vi "MagnetoGUI_Vorschlag.vi"() -> ()   [LabVIEW 2016]
uses:
  controls/GUI Parameter.ctl
  controls/State.ctl
  controls/Data.ctl
panel:
  out "Tab Control":T1(tab)
  in  "Taster Einstellungen":bool
  in  "Anzahl Messpunkte Neukurve":i8=16 min=10 max=30 step=1
  out "Hystereseschleife und Neukurve / Preview":cluster{dbl[], dbl[]}[](graph) caption="XY Graph"
  in  "Plot_Speichern":bool
  out "Status":bool
  in  "Start Button":bool
  in  "Maximieren":bool
  in  "GUI Parameter":T2={"Eisenquerschnitt [mm^2]"=45.0, "Wirksame Länge [cm]"=94.0, "Primärwindungszahl"=700.0, "Sekundärwindungszahl"=700.0, "Messwiderstand [Ohm]"=1.0, "Spannungsteilerverhaeltnis (1/x)"=1.0, "Probenbezeichnung"="", "Dichte des Eisens [g/cm^3]"=7.0, "magn. Flussdichte [T]"=2.0, "Frequenz [Hz]"=50.0, "Namen"="", "Gruppe"=""}
  in  "Neukurve Messen?":bool
  in  "Minimale Spannung [V]":dbl=0.01
  in  "Maximale Spannung [V]":dbl=10.0
  out "Faktor2":dbl
  out "Faktor1":dbl
  out "Theo. Primärwindungszahl":dbl
  in  "Taster Hauptansicht":bool
  in  "VISA Name Oszilloscope":refnum<visa-resource-name>="USB0::0x0957::0x179B::MY54313507::INSTR"
  in  "VISA Name Frequenzgen.":refnum<visa-resource-name>="USB0::0x0957::0x0407::MY44043889::INSTR"
  in  "Anzahl der Oszi-Messpunkte":i32=6000
  in  "Excel Export":bool
  out "Gruppe":string
  out "Namen":string
  out "Frequenz [Hz]":dbl
  out "magn. Flussdichte [T]":dbl
  out "Dichte des Eisens [g/cm^3]":dbl
  out "Probenbezeichnung":string
  out "Spannungsteilerverhältnis (1/x)":dbl
  out "Messwiderstand [Ohm]":dbl
  out "Sekundärwindungszahl":dbl
  out "Primärwindungszahl":dbl
  out "Wirksame Länge [cm]":dbl
  out "Eisenquerschnitt [mm^2]":dbl
  in  "Minimieren":bool
  in  "Ansicht_Speichern":bool
  out "Hystereseschleife und Neukurve":cluster{dbl[], dbl[]}[](graph) caption="XY Graph"
  in  "Plot_Speichern 2":bool
  out "Datum/Uhrzeit":timestamp format="%<%H:%M\n%d/%m/%y>T"
  out "Hystereseverluste [W]":dbl
  # "Laborversuch: Magnetische Eigenschaften"
  # "Laborversuch: Magnetische Eigenschaften"
  # "Oszilloskop Messpunkte"
  # "System Setup"
  # "Frequenzgenerator"
  # "Strombegrenzung"
  # "Anzeige der berechneten Größen"
  # "Maximal Strom [A]"
  # "Laborversuch: Magnetische Eigenschaften"
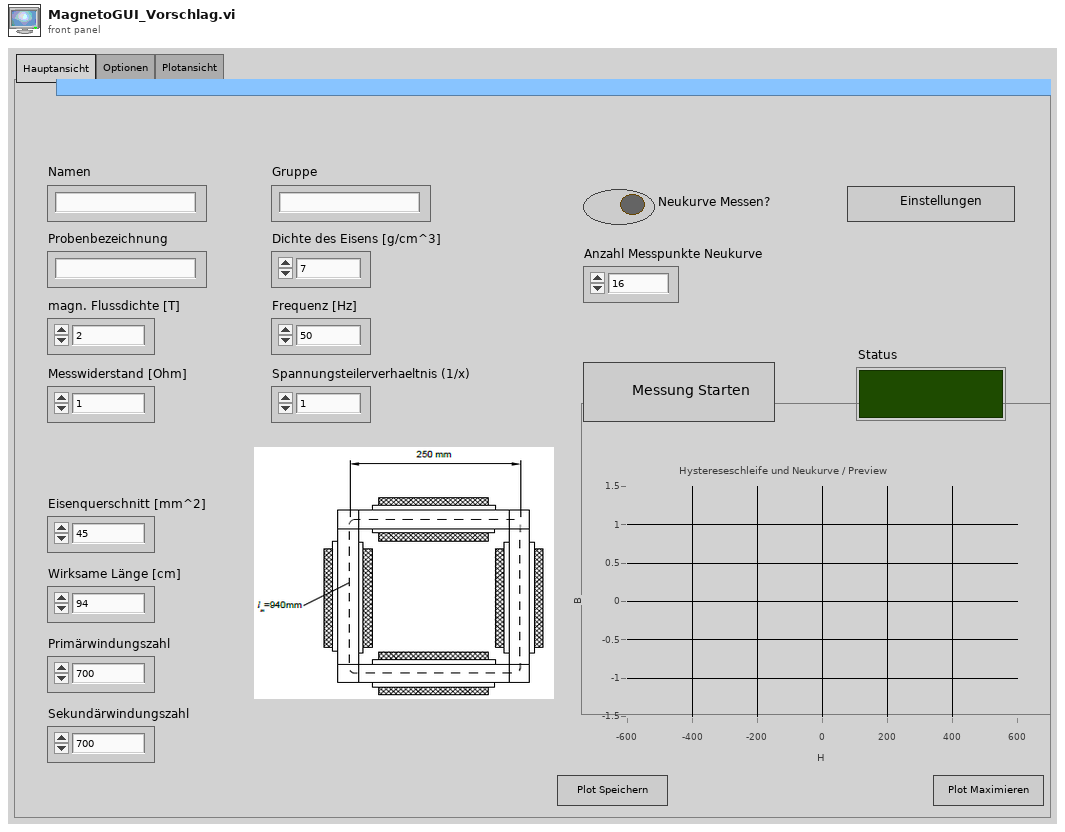
[diagram p1: front panel]
types:
  T1 = enum32{"Hauptansicht", "Optionen", "Plotansicht"}
  T2 = typedef "GUI Parameter.ctl" = cluster{"Eisenquerschnitt [mm^2]":dbl, "Wirksame Länge [cm]":dbl, "Primärwindungszahl":dbl, "Sekundärwindungszahl":dbl, "Messwiderstand [Ohm]":dbl, "Spannungsteilerverhaeltnis (1/x)":dbl, "Probenbezeichnung":string, "Dichte des Eisens [g/cm^3]":dbl, "magn. Flussdichte [T]":dbl, "Frequenz [Hz]":dbl, "Namen":string, "Gruppe":string}
  T3 = typedef "Data.ctl" = cluster{"GUI Einstellungen":cluster{"Spannungsabweichung":dbl, "Maximale Spannung FG":dbl, "Faktor1":dbl, "Faktor2":dbl, "Theoretische Primärwindungszahl":dbl, "Anzahl der Messpunkte":i32, "VISA Name Oszilloscope":refnum<visa-resource-name>, "VISA Name Frequenzgenerator":refnum<visa-resource-name>, "Minimale Spannung FG":dbl, "Pfad für Messwerte und Plots":path}, "GUI data":cluster{"Eisenquerschnitt [mm^2]":dbl, "Wirksame Länge [cm]":dbl, "Primärwindungszahl":dbl, "Sekundärwindungszahl":dbl, "Messwiderstand [Ohm]":dbl, "Spannungsteilerverhaeltnis (1/x)":dbl, "Probenbezeichnung":string, "Dichte des Eisens [g/cm^3]":dbl, "magn. Flussdichte [T]":dbl, "Frequenz [Hz]":dbl, "Namen":string, "Gruppe":string}, "B - Neukurve Array":dbl[], "H - Neukurve Array":dbl[], "Messung Hystereseschleife":cluster{"b_gew":dbl, "b_kor":dbl, "hys_verluste":dbl, "punkte":i32, "B - Hysterese Array":dbl[], "H - Hysterese Array":dbl[]}, "Messung Neukurve":cluster{"Neukurve Messen?":bool, "Anzahl Messpunkte Neukurve":i8}, "Globale Variablen":cluster{"merker1":bool, "merker2":bool, "merker3":bool, "merker4":bool, "merker5":bool, "merker6":bool, "merker7":bool, "merker8":bool, "merker9":bool, "bmax1":dbl, "bmin1":dbl, "bmax2":dbl, "bmin2":dbl, "spg_abw":dbl, "Tatsächliche Flussdichte":dbl, "Tatsächliche Anzahl Punkte":dbl, "hmax1":dbl, "hmin1":dbl, "hmax2":dbl}}
  T4 = typedef "State.ctl" = enum16{"Initialisieren", "Warten auf Event", "Starten der Messung", "Initialisieren Hardware", "Flussdichte Einstellen", "Chk Flussdichte Anpassung", "Messung Hystereseschleife", "Entmagnetisieren", "Messung Neukurve", "Messung Kommutierungskurve", "Ausgabe Diagramm", "Ende", "Plot aufnehmen", "Ansicht speichern", "Excel Export"}
  T5 = cluster{"Spannungsabweichung":dbl, "Maximale Spannung FG":dbl, "Faktor1":dbl, "Faktor2":dbl, "Theoretische Primärwindungszahl":dbl, "Anzahl der Messpunkte":i32, "VISA Name Oszilloscope":refnum<visa-resource-name>, "VISA Name Frequenzgenerator":refnum<visa-resource-name>, "Minimale Spannung FG":dbl, "Pfad für Messwerte und Plots":path}
  T6 = cluster{"Eisenquerschnitt [mm^2]":dbl, "Wirksame Länge [cm]":dbl, "Primärwindungszahl":dbl, "Sekundärwindungszahl":dbl, "Messwiderstand [Ohm]":dbl, "Spannungsteilerverhaeltnis (1/x)":dbl, "Probenbezeichnung":string, "Dichte des Eisens [g/cm^3]":dbl, "magn. Flussdichte [T]":dbl, "Frequenz [Hz]":dbl, "Namen":string, "Gruppe":string}
  T7 = cluster{"merker1":bool, "merker2":bool, "merker3":bool, "merker4":bool, "merker5":bool, "merker6":bool, "merker7":bool, "merker8":bool, "merker9":bool, "bmax1":dbl, "bmin1":dbl, "bmax2":dbl, "bmin2":dbl, "spg_abw":dbl, "Tatsächliche Flussdichte":dbl, "Tatsächliche Anzahl Punkte":dbl, "hmax1":dbl, "hmin1":dbl, "hmax2":dbl}
  T8 = cluster{"b_gew":dbl, "b_kor":dbl, "hys_verluste":dbl, "punkte":i32, "B - Hysterese Array":dbl[], "H - Hysterese Array":dbl[]}
  T9 = cluster{"H - Hysterese Array":dbl[], "B - Hysterese Array":dbl[]}
  T10 = cluster{"H - Neukurve Array":dbl[], "B - Neukurve Array":dbl[]}
  T11 = cluster{"H - Neukurve Array":dbl[], "B - Neukurve Array":dbl[]}[]
  T12 = typedef "imagedata.ctl" = cluster{"image type":i32, "image depth":i32, "image":u8[], "mask":u8[], "colors":u32[], "Rectangle":cluster{"left":i16, "top":i16, "right":i16, "bottom":i16}}
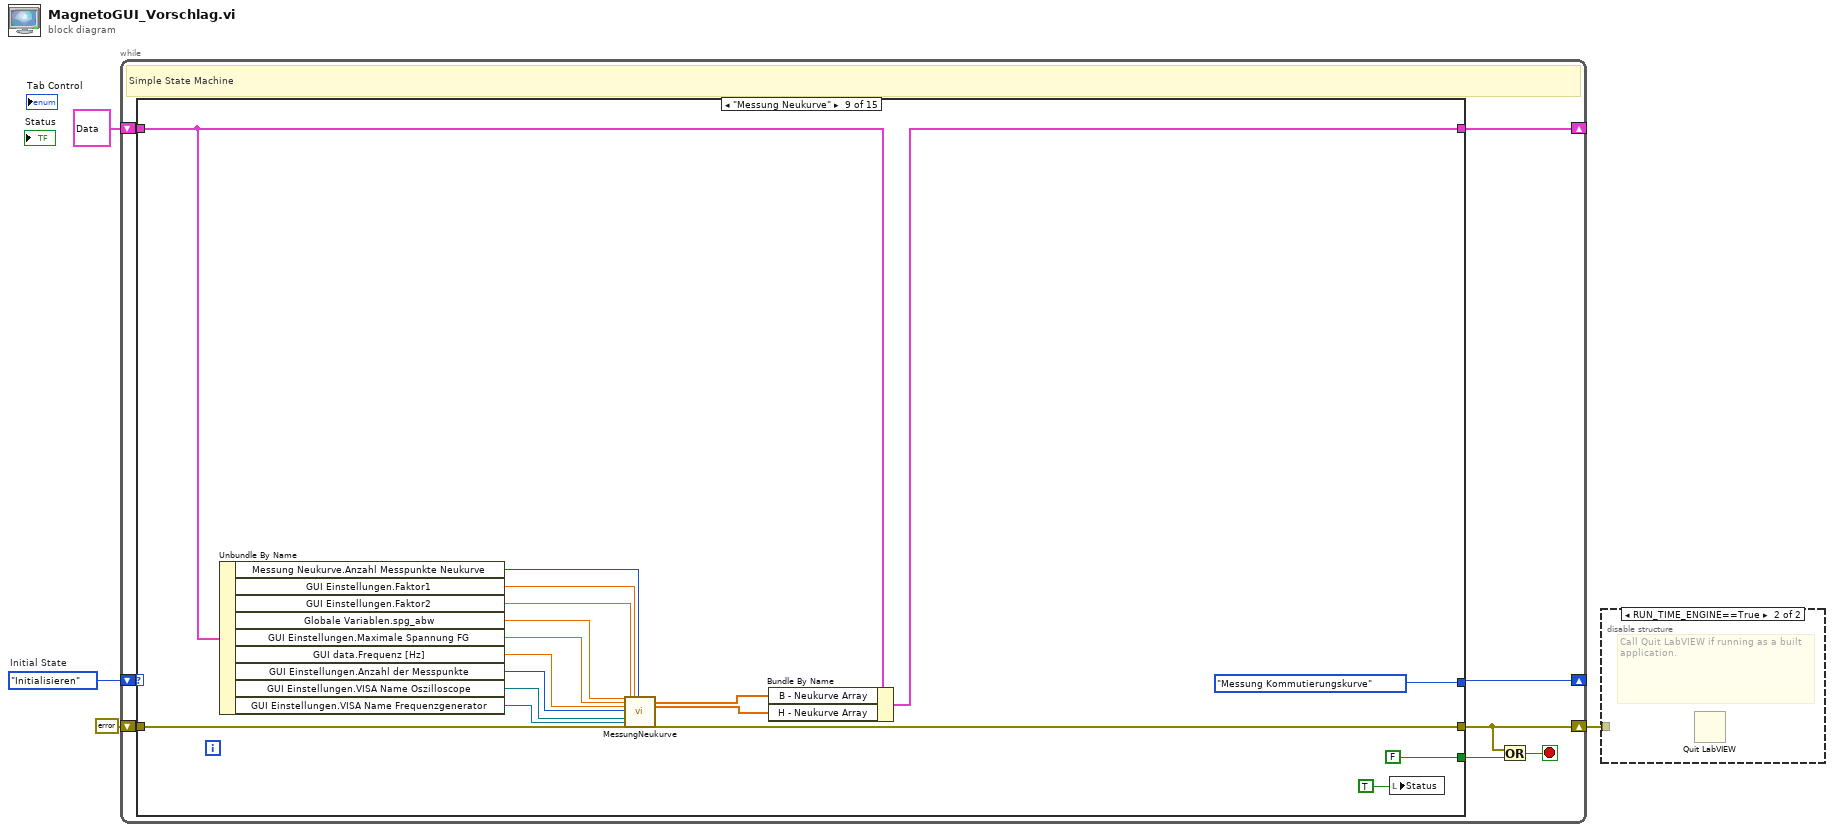
[diagram p0: block diagram]
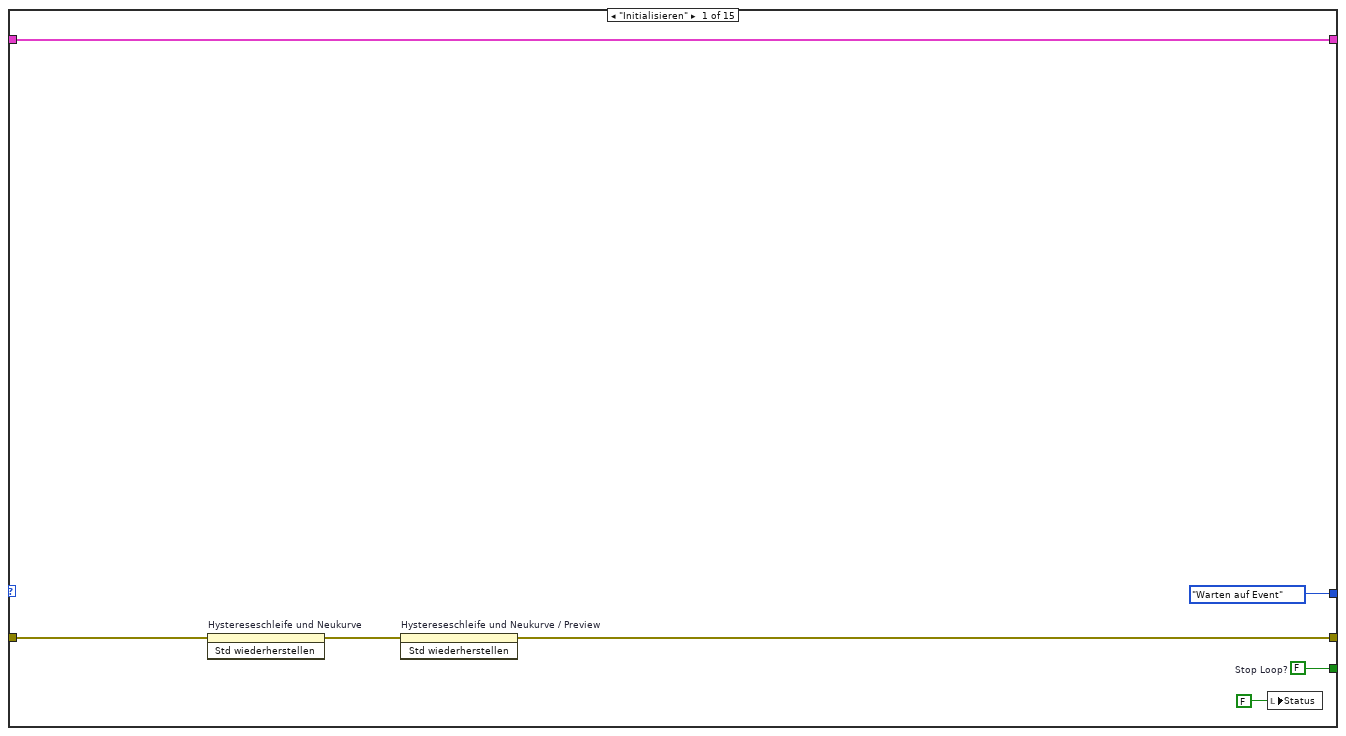
[diagram p2: hidden frame]
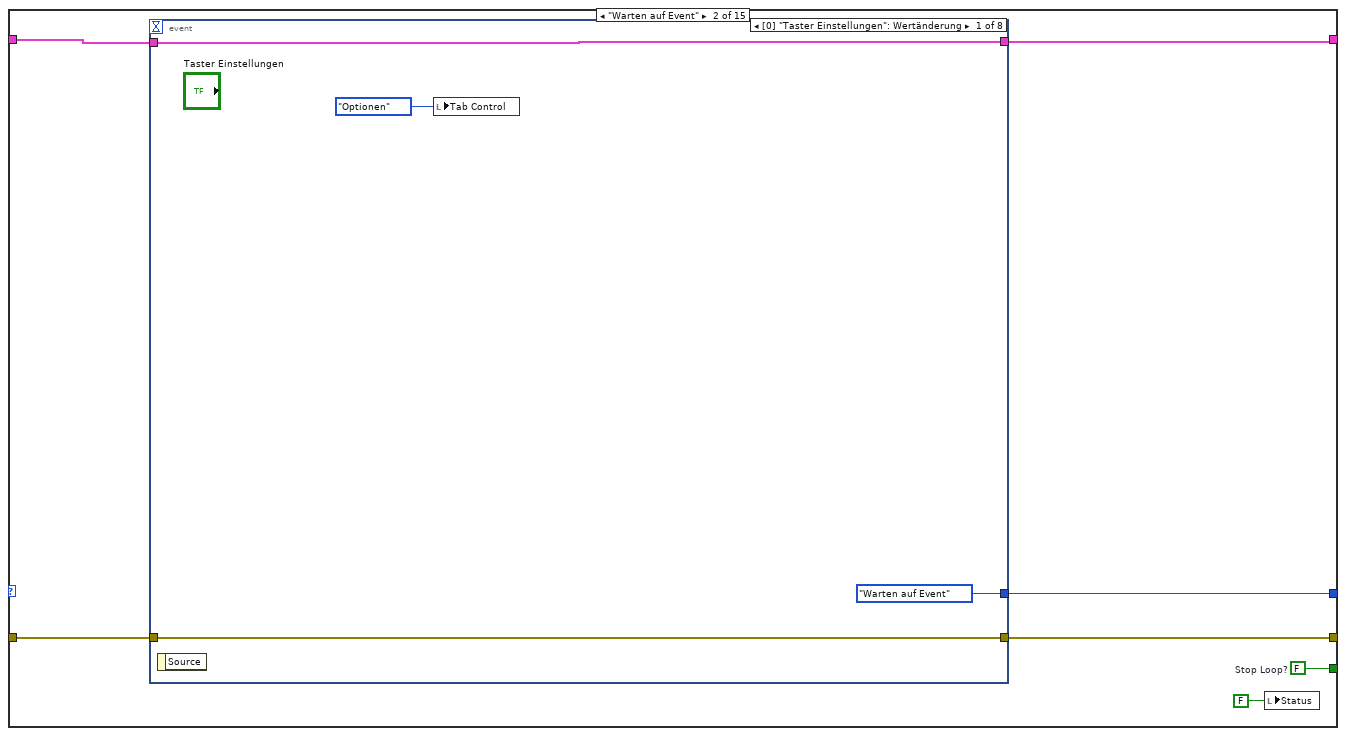
[diagram p3: hidden frame]
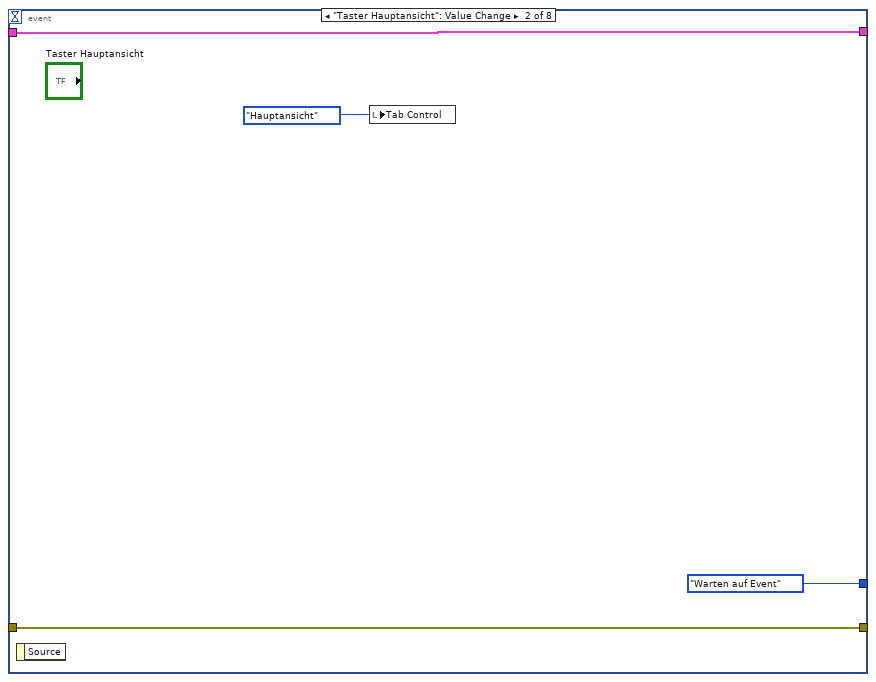
[diagram p4: hidden frame]
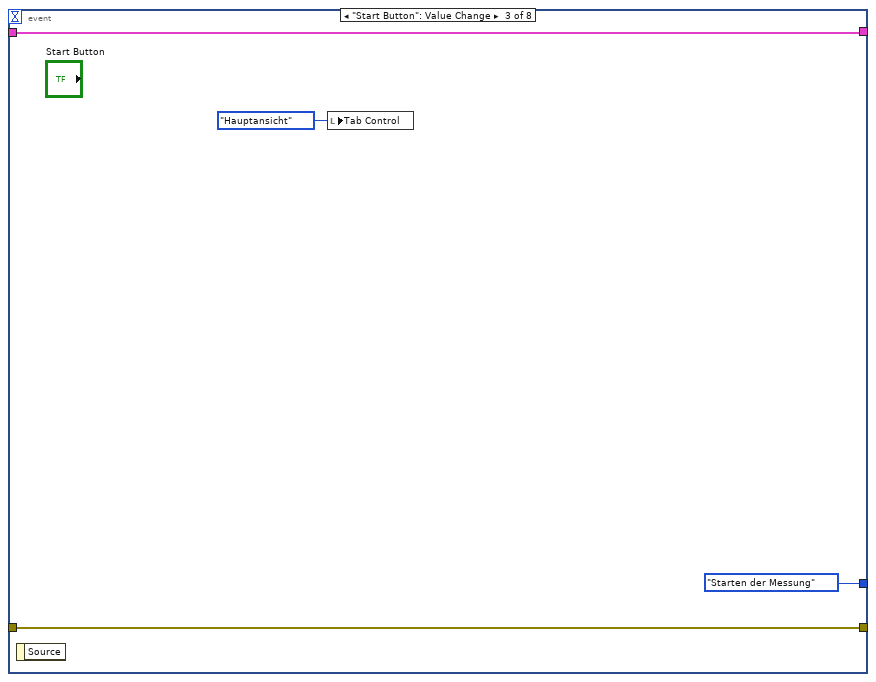
[diagram p5: hidden frame]
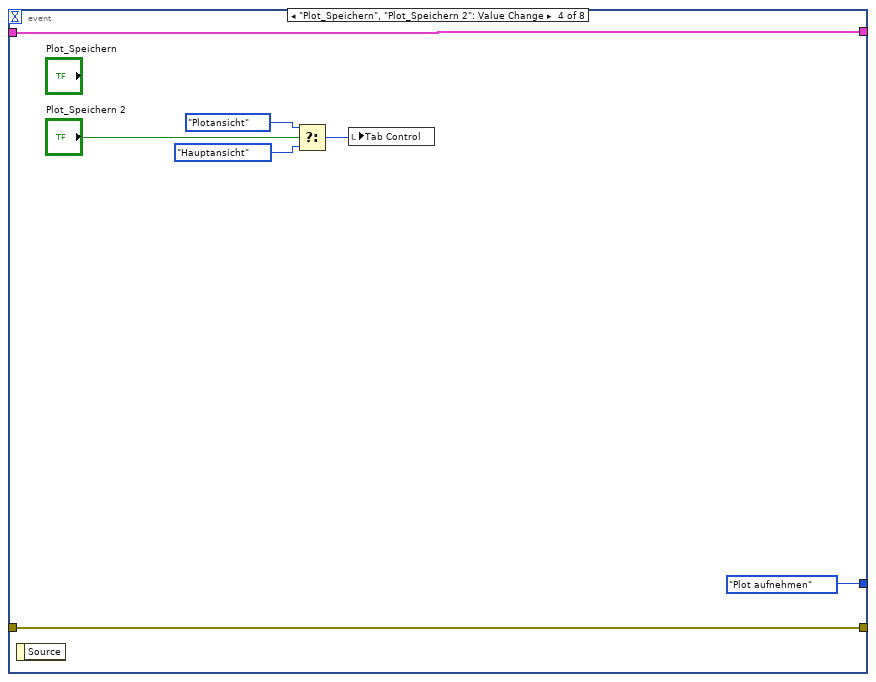
[diagram p6: hidden frame]
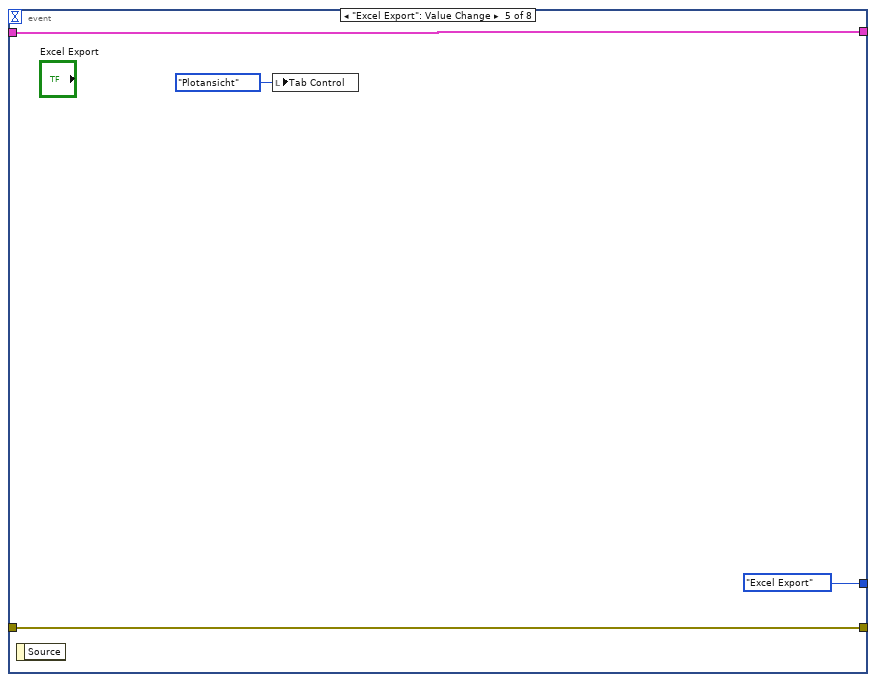
[diagram p7: hidden frame]
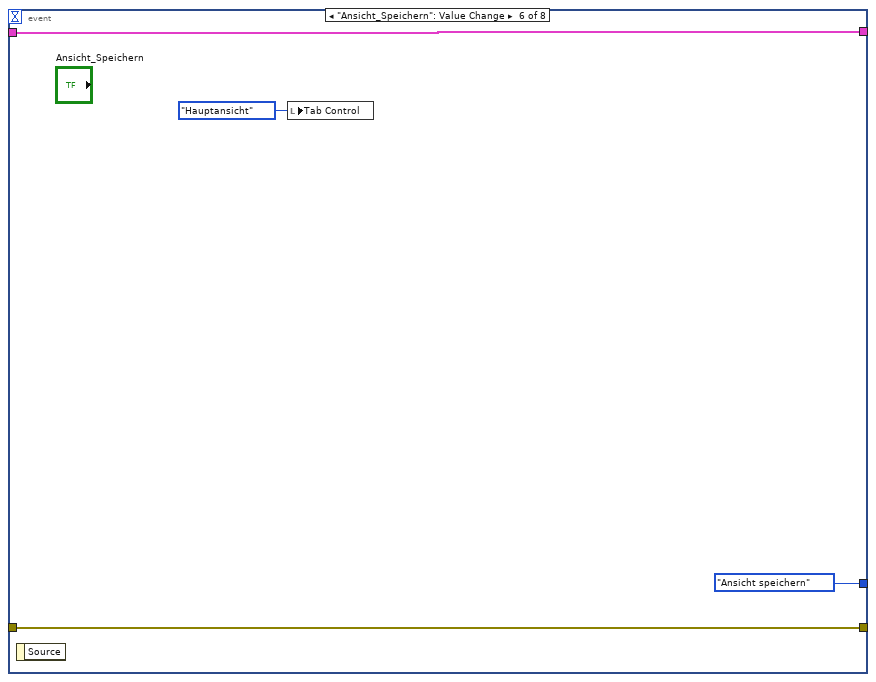
[diagram p8: hidden frame]
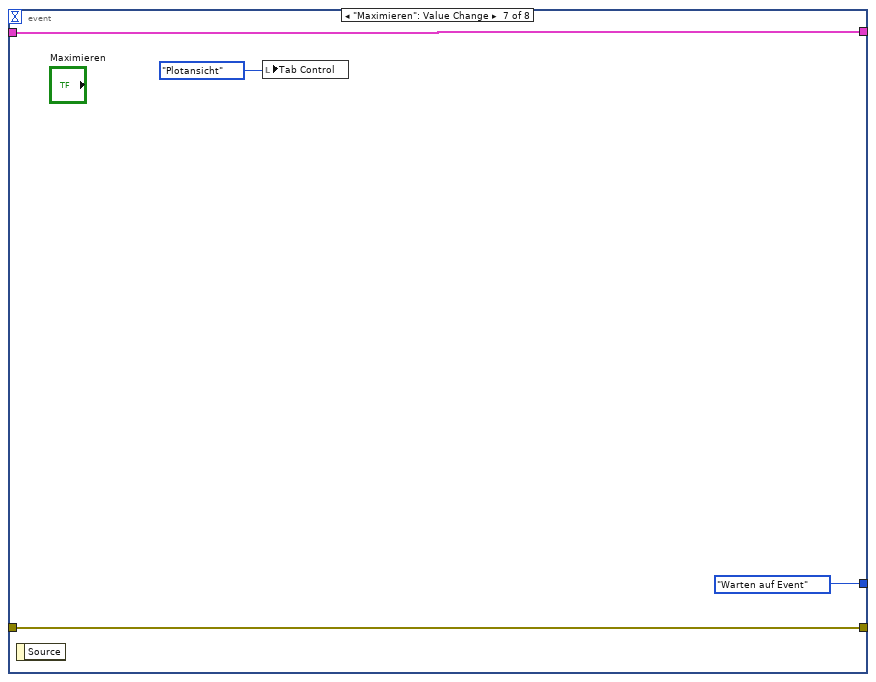
[diagram p9: hidden frame]
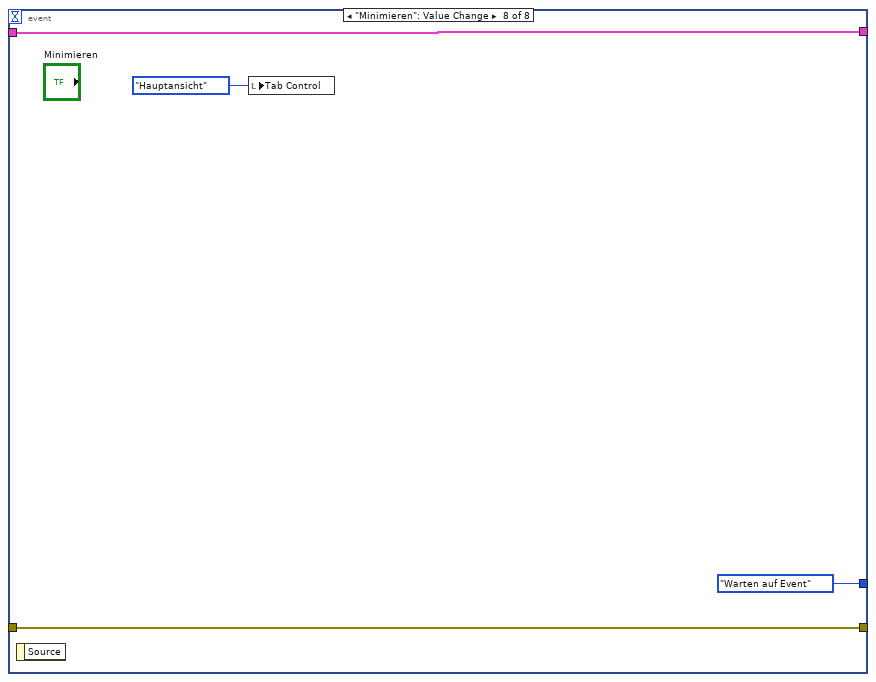
[diagram p10: hidden frame]
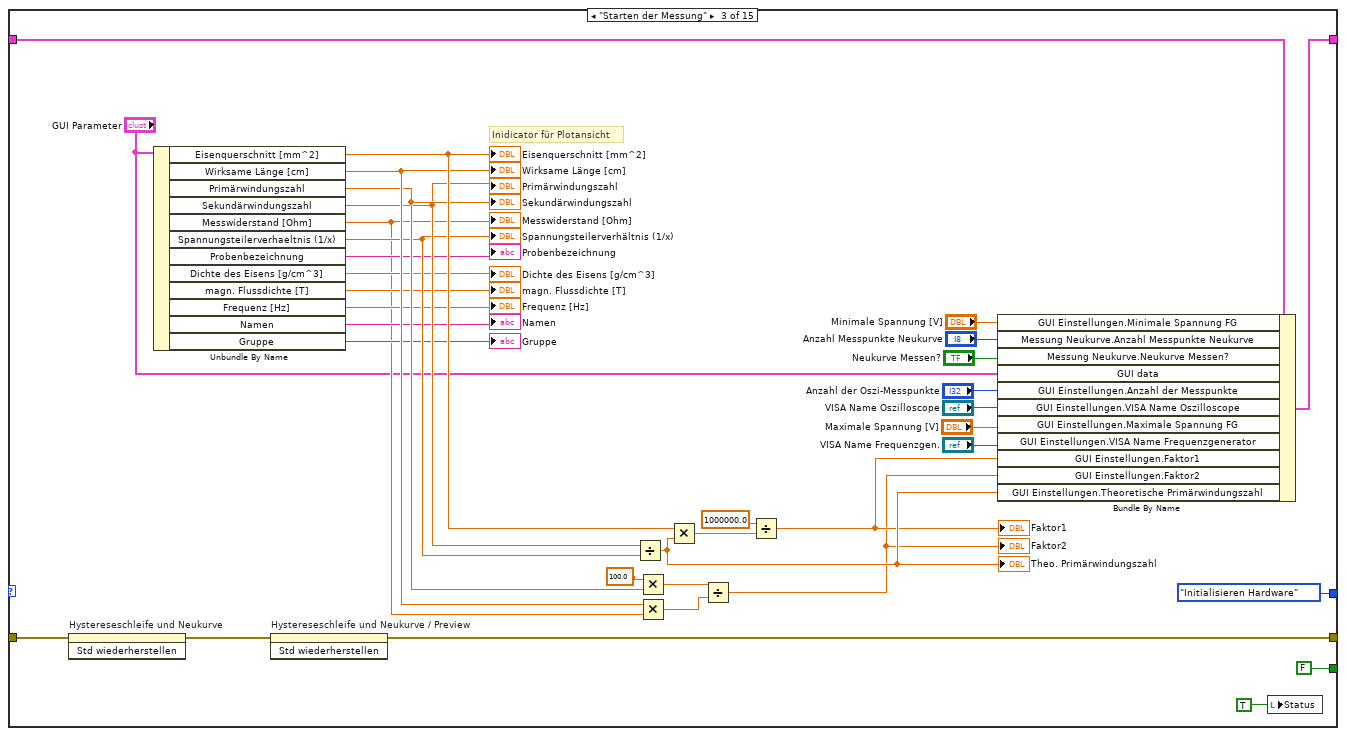
[diagram p11: hidden frame]
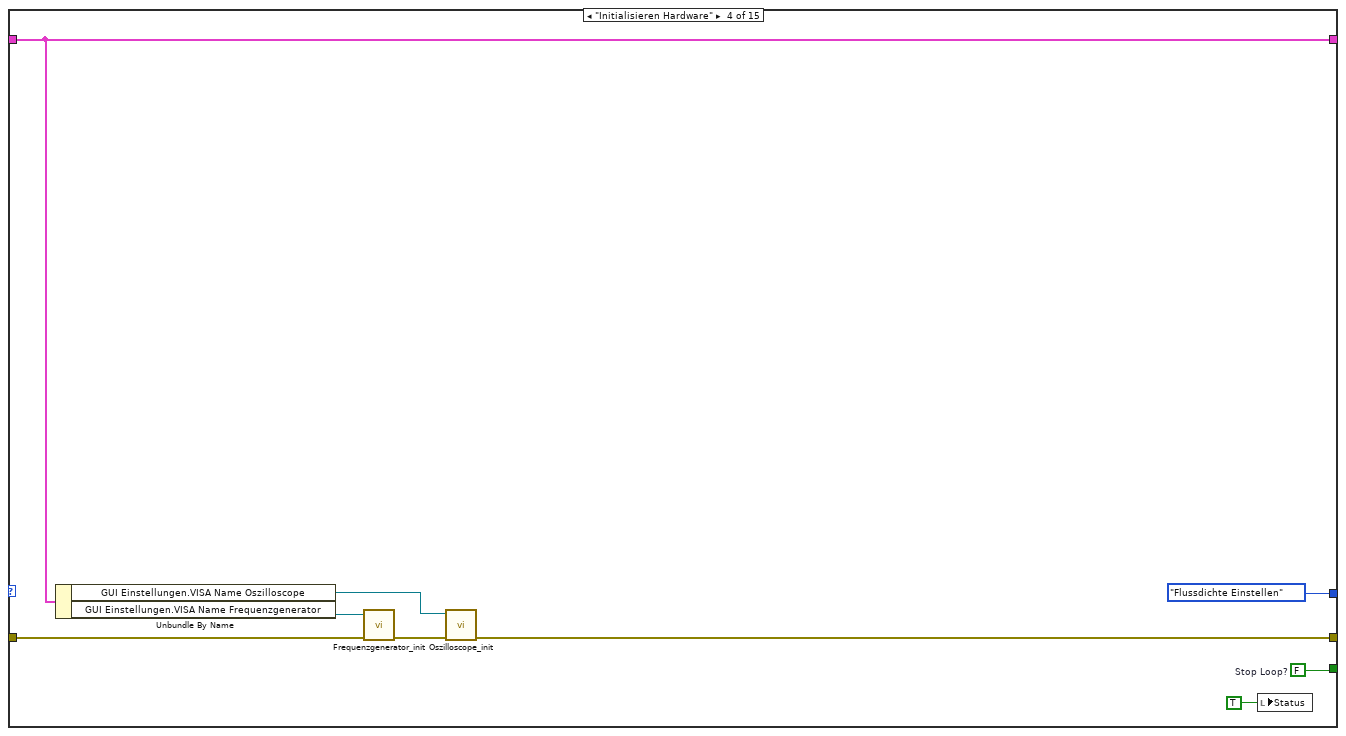
[diagram p12: hidden frame]
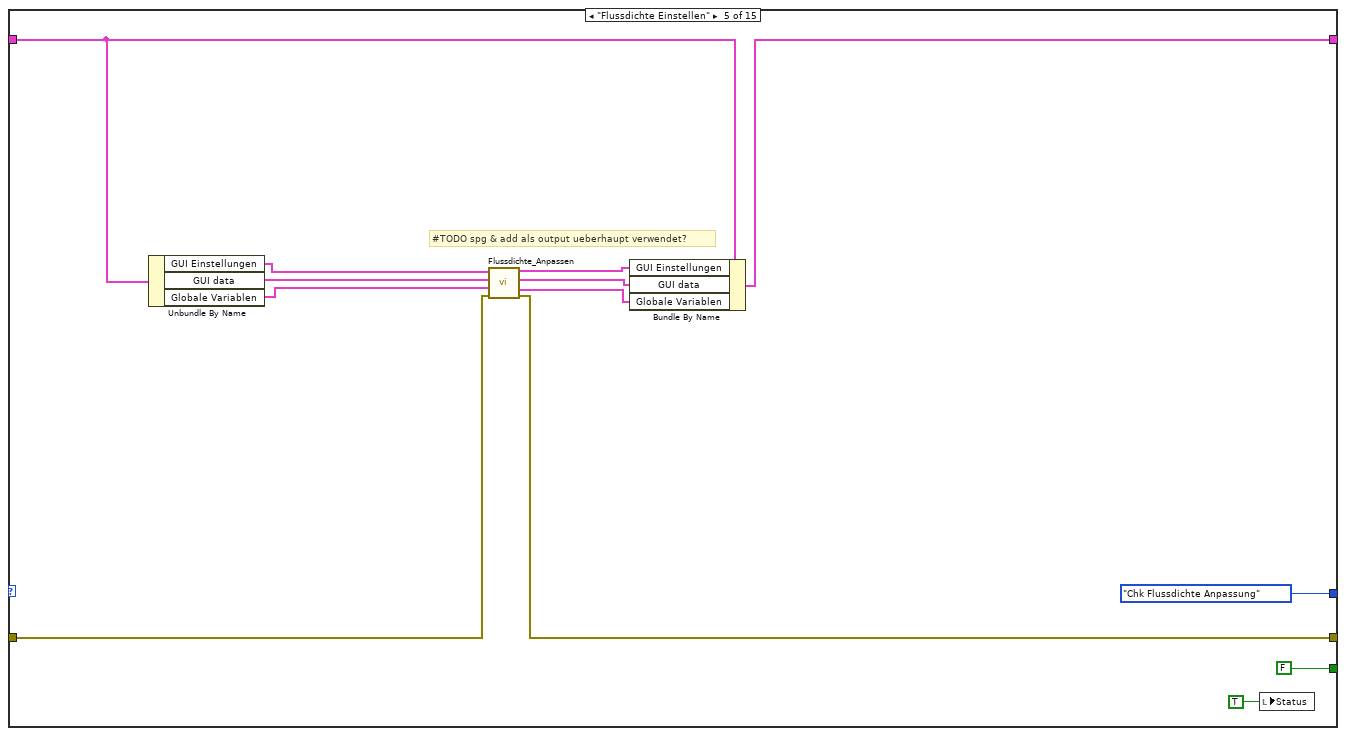
[diagram p13: hidden frame]
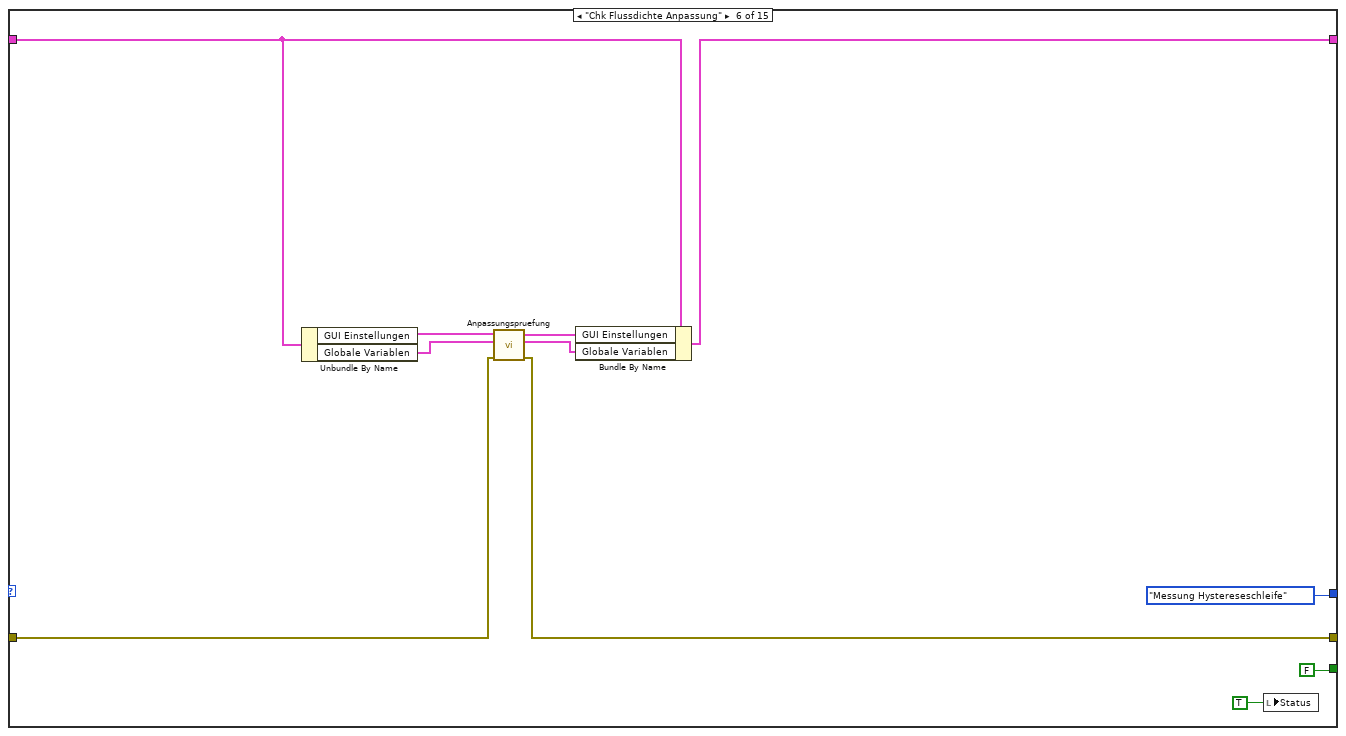
[diagram p14: hidden frame]
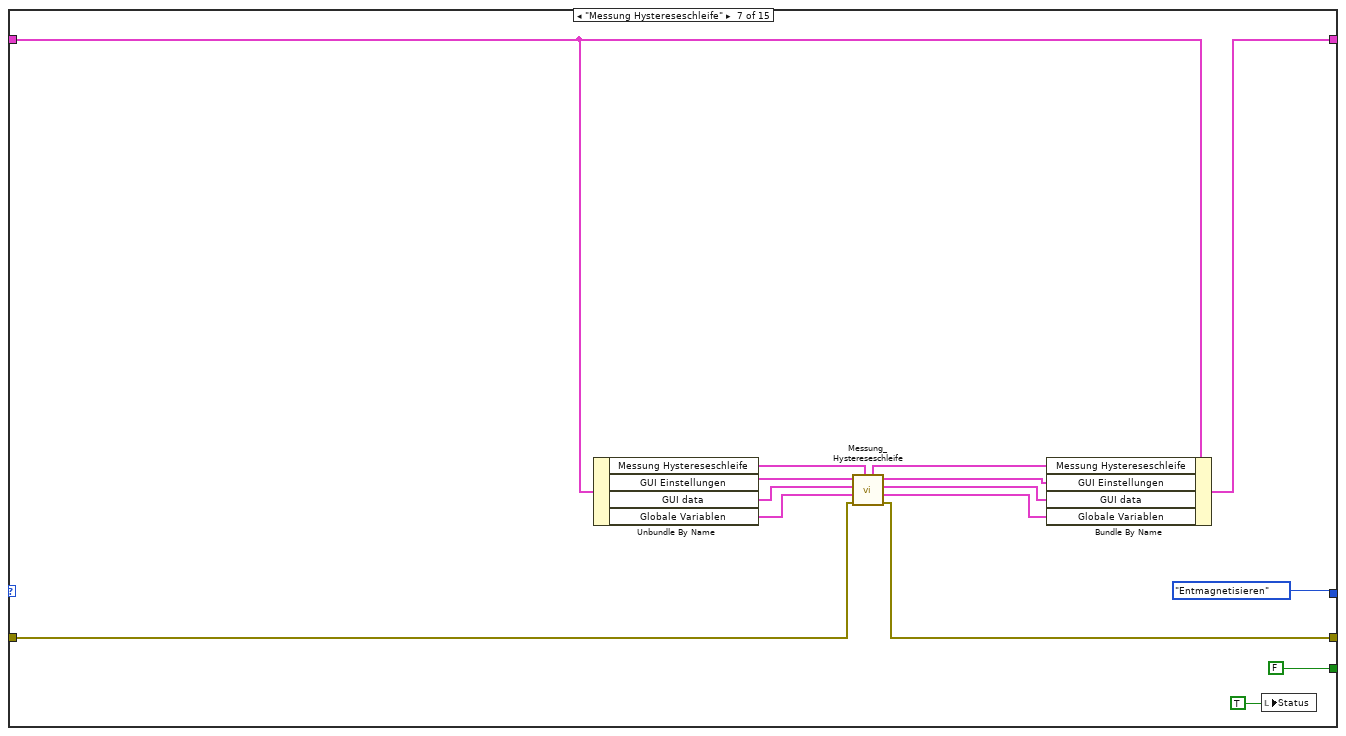
[diagram p15: hidden frame]
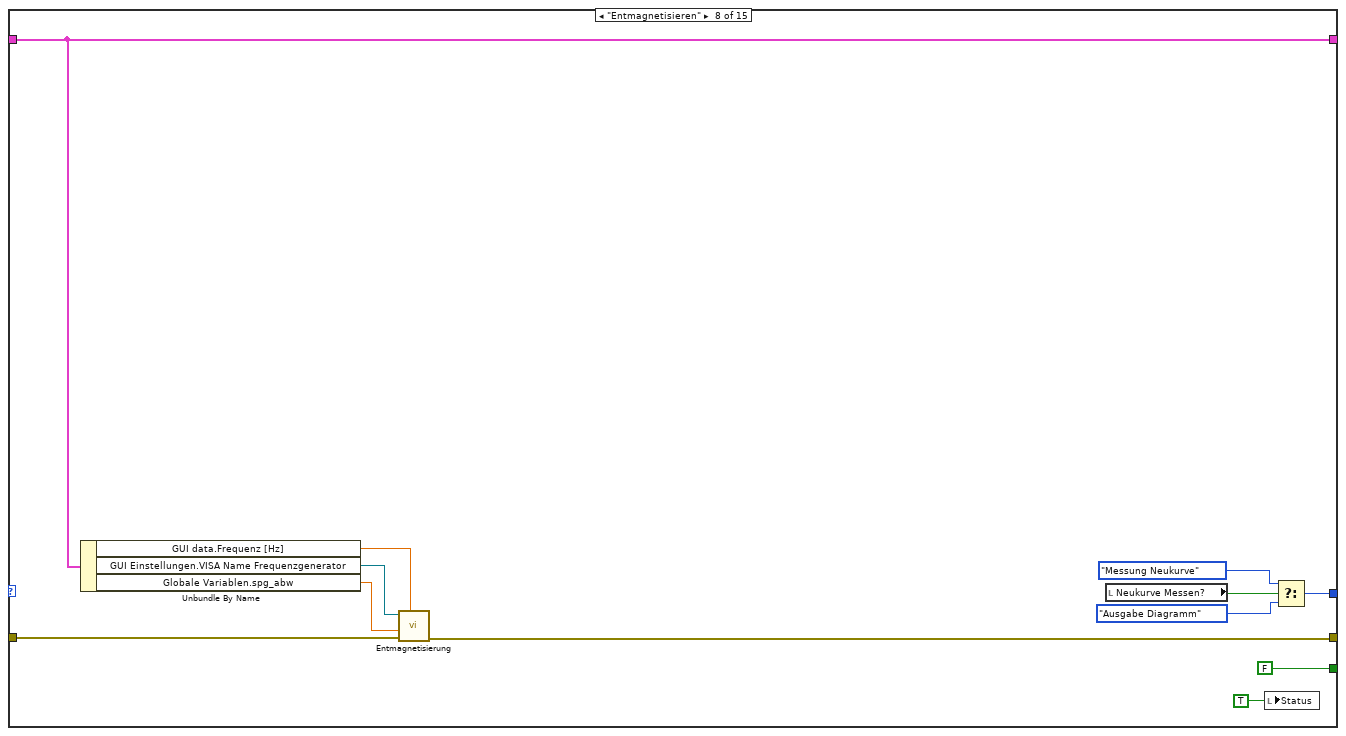
[diagram p16: hidden frame]
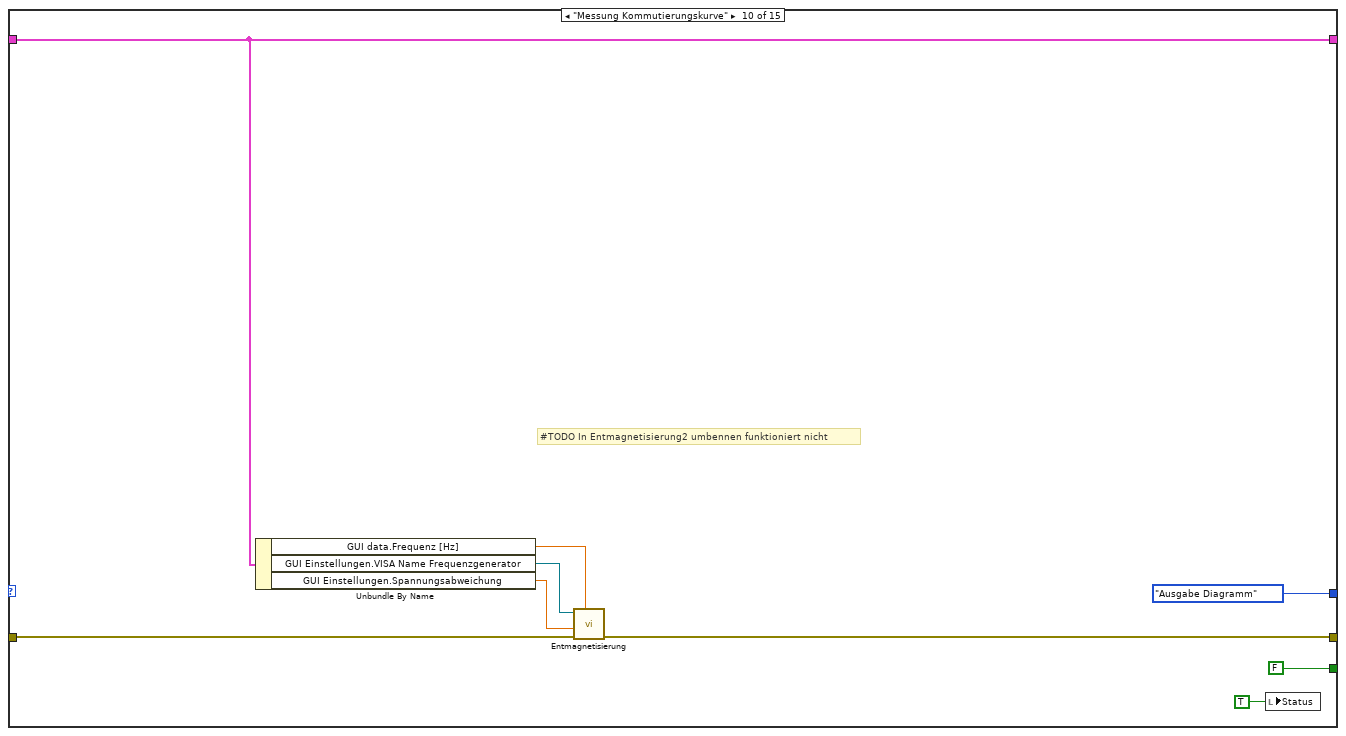
[diagram p17: hidden frame]
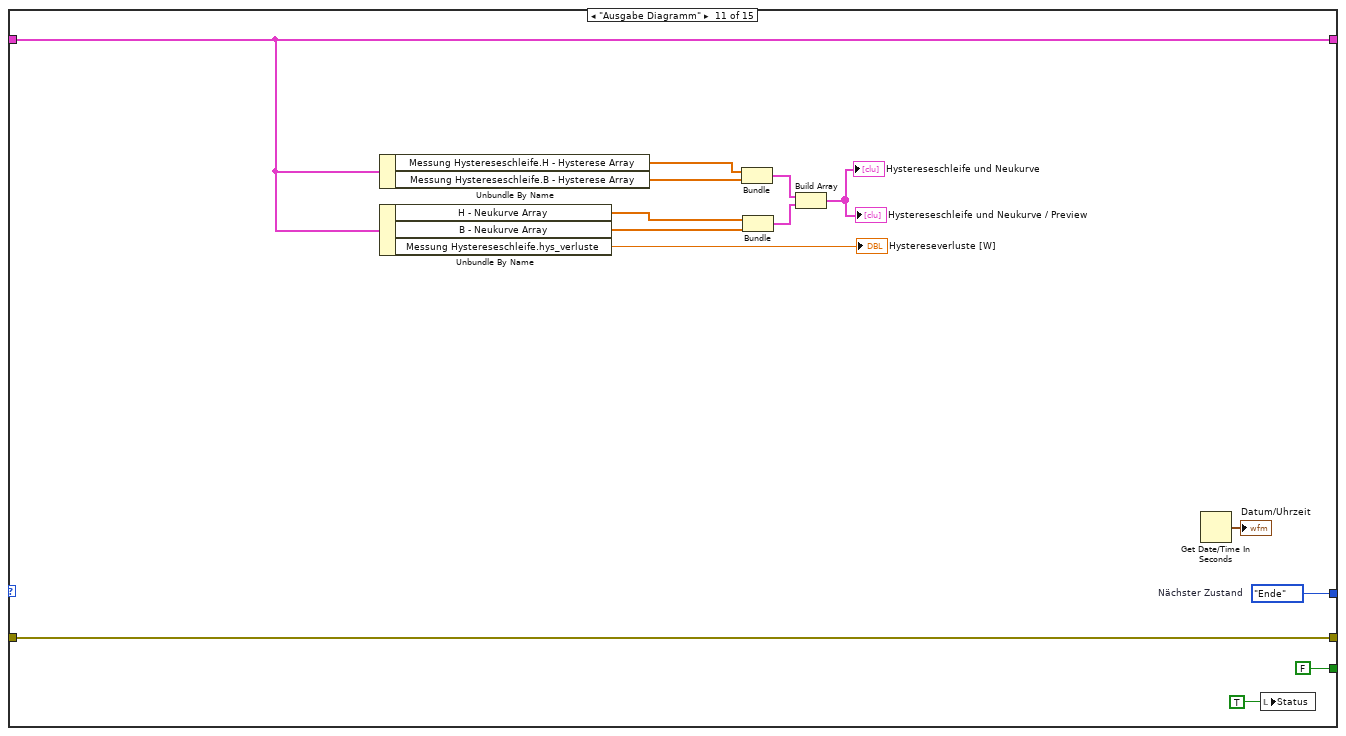
[diagram p18: hidden frame]
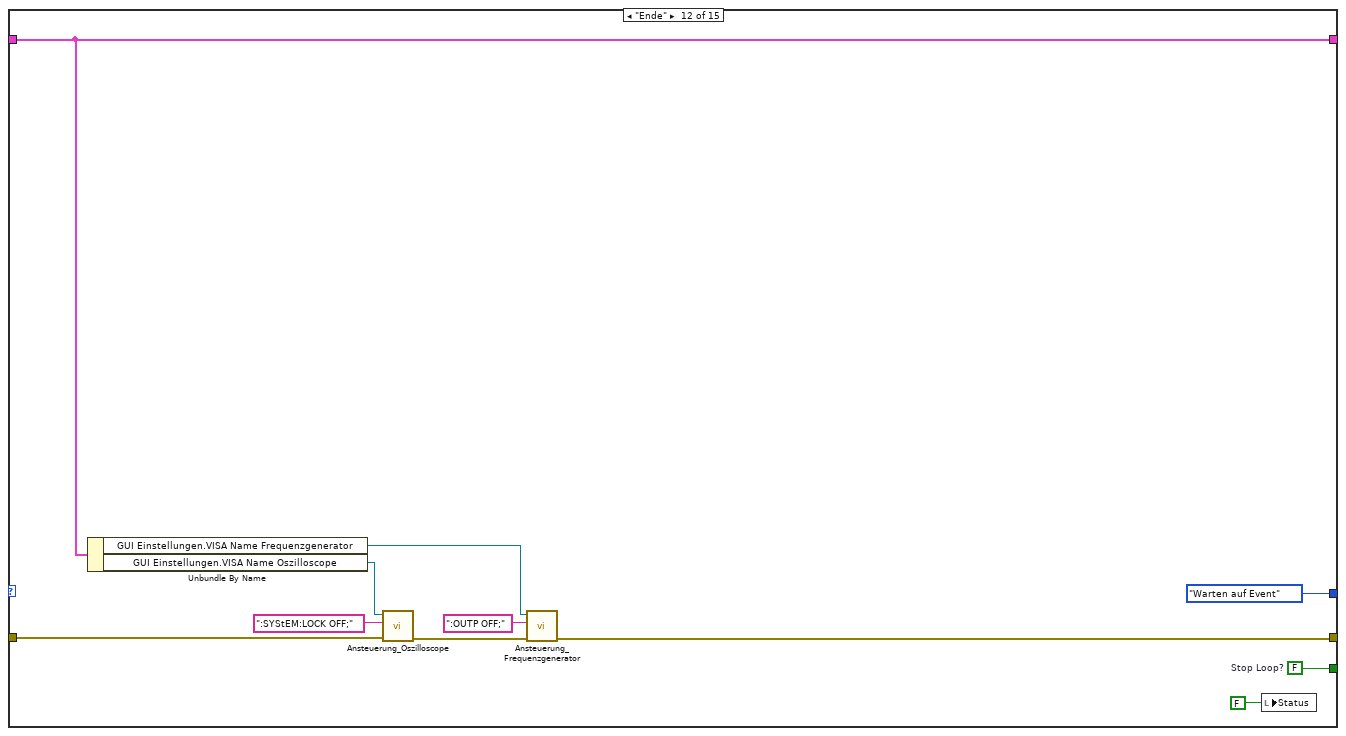
[diagram p19: hidden frame]
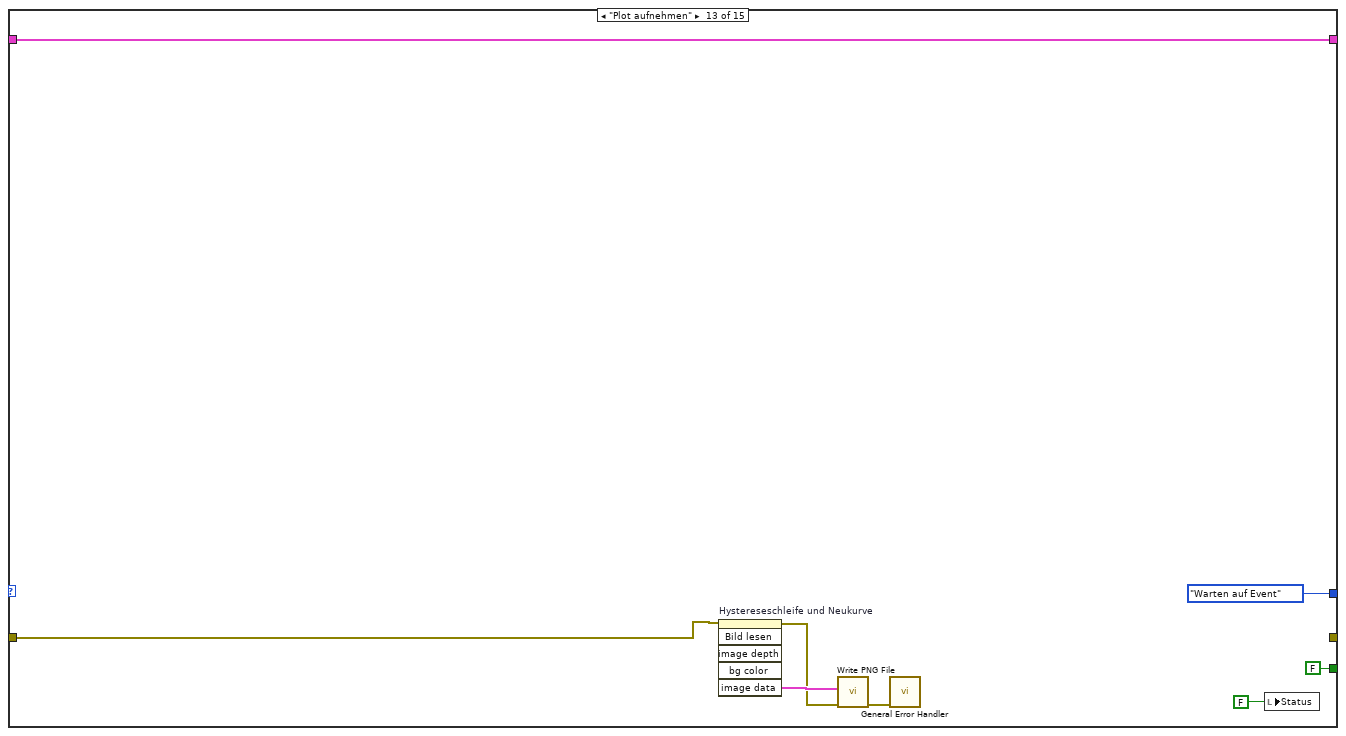
[diagram p20: hidden frame]
diagram:
  w4 = State."Initialisieren"  # Initial State
  n1 = while {
    shift-right: [w11] -> _
    shift-left: w4 -> [w12]
    shift-right: [w9] -> _
    shift-left: T3 {"GUI Einstellungen"={"Spannungsabweichung"=0.0, "Maximale Spannung FG"=0.0, "Faktor1"=0.0, "Faktor2"=0.0, "Theoretische Primärwindungszahl"=0.0, "Anzahl der Messpunkte"=0, "VISA Name Oszilloscope"="", "VISA Name Frequenzgenerator"="", "Minimale Spannung FG"=0.0, "Pfad für Messwerte und Plots"=path ""}, "GUI data"={"Eisenquerschnitt [mm^2]"=0.0, "Wirksame Länge [cm]"=0.0, "Primärwindungszahl"=0.0, "Sekundärwindungszahl"=0.0, "Messwiderstand [Ohm]"=0.0, "Spannungsteilerverhaeltnis (1/x)"=0.0, "Probenbezeichnung"="", "Dichte des Eisens [g/cm^3]"=0.0, "magn. Flussdichte [T]"=0.0, "Frequenz [Hz]"=0.0, "Namen"="", "Gruppe"=""}, "B - Neukurve Array"=[], "H - Neukurve Array"=[], "Messung Hystereseschleife"={"b_gew"=0.0, "b_kor"=0.0, "hys_verluste"=0.0, "punkte"=0, "B - Hysterese Array"=[0.0, 0.0], "H - Hysterese Array"=[0.0, 0.0]}, "Messung Neukurve"={"Neukurve Messen?"=FALSE, "Anzahl Messpunkte Neukurve"=16}, "Globale Variablen"={"merker1"=FALSE, "merker2"=FALSE, "merker3"=FALSE, "merker4"=FALSE, "merker5"=FALSE, "merker6"=FALSE, "merker7"=FALSE, "merker8"=FALSE, "merker9"=FALSE, "bmax1"=0.0, "bmin1"=0.0, "bmax2"=0.0, "bmin2"=0.0, "spg_abw"=0.0, "Tatsächliche Flussdichte"=0.0, "Tatsächliche Anzahl Punkte"=0.0, "hmax1"=0.0, "hmin1"=0.0, "hmax2"=0.0}} ("Data") -> [w10]
    shift-right: [w5] -> w1
    shift-left: errorcluster {"status"=FALSE, "code"=0, "source"=""} ("error constant") -> [w8]
    stop <- w6 stop-if-true
    # "Simple State Machine"
    n2 = case shown="\"Messung Neukurve\"" w12 {
      tunnel: [State."Warten auf Event" ("Next State") w26 State."Initialisieren Hardware" ("Next State") State."Flussdichte Einstellen" ("Next State") State."Chk Flussdichte Anpassung" ("Next  State") State."Messung Hystereseschleife" ("Next  State") State."Entmagnetisieren" ("(Value Not Used)") w147 State."Messung Kommutierungskurve" ("(Value Not Used)") State."Ausgabe Diagramm" ("(Value Not Used)") w196 State."Warten auf Event" ("Next  State") State."Warten auf Event" ("Next  State") State."Warten auf Event" ("Next  State") State."Warten auf Event" ("Next  State")] -> w11
      tunnel: [w18 w25 FALSE ("Stop Loop?") w99 FALSE ("Stop Loop?") FALSE ("Stop Loop?") FALSE ("Stop Loop?") FALSE ("Stop Loop?") FALSE ("Stop Loop?") FALSE ("Stop Loop?") FALSE ("Stop Loop?") w209 FALSE ("Stop Loop?") FALSE ("Stop Loop?") FALSE ("Stop Loop?")] -> w7
      tunnel: w10 -> [w17 w24 w75 w105 w114 w126 w133 w156 w163 w177 w191 w207 w217 w225 w232]
      tunnel: [w17 w23 w76 w105 w113 w125 w144 w156 w167 w177 w191 w207 w217 w225 w232] -> w9
      tunnel: w8 -> [w16 w22 w95 w104 w115 w121 w132 w155 w173 w179 w195 w208 w215 w221 w230]
      tunnel: [w14 w21 w77 w102 w109 w122 w134 w154 w172 w178 w195 w202 _ _ w229] -> w5
      frame "Initialisieren" {
        w18 = FALSE  # Stop Loop?
        n3 = invoke on="Hystereseschleife und Neukurve" class="XYGraph (strikt)" method="Std wiederherstellen"(error in=w16) -> (error out=w15:errorcluster)  [unwired: 2 in, 2 out]
        n4 = invoke on="Hystereseschleife und Neukurve / Preview" class="XYGraph (strikt)" method="Std wiederherstellen"(error in=w15) -> (error out=w14:errorcluster)  [unwired: 2 in, 2 out]
        n5 = local write "Status"(FALSE ("Status")) -> ()
      }
      frame "Warten auf Event" {
        w25 = FALSE  # Stop Loop?
        n6 = event shown="[0] \"Taster Einstellungen\": Wertänderung" {
          selector: _ -> [_ _ _ _ _ _ _ _]
          dyn-events: _ -> [_ _ _ _ _ _ _ _]
          timeout: _ -> [_ _ _ _ _ _ _ _]
          tunnel: [State."Warten auf Event" State."Warten auf Event" ("Next State") State."Starten der Messung" ("Next State") State."Plot aufnehmen" ("Next State") State."Excel Export" ("Next State") State."Ansicht speichern" ("Next State") State."Warten auf Event" ("Next State") State."Warten auf Event" ("Next State")] -> w26
          tunnel: w24 -> [w30 w34 w36 w45 w49 w53 w55 w61]
          tunnel: [w30 w34 w36 w45 w49 w53 w55 w61] -> w23
          tunnel: w22 -> [w29 w33 w37 w39 w46 w50 w56 w60]
          tunnel: [w29 w33 w37 w39 w46 w50 w56 w60] -> w21
          event "Taster Einstellungen": Value Change {
            n7 = event-data() -> ()  [unwired: 1 in, 1 out]
            n8 = local write "Tab Control"(T1."Optionen" ("Tab Control")) -> ()
          }
          event "Taster Hauptansicht": Value Change {
            n9 = event-data() -> ()  [unwired: 1 in, 1 out]
            n10 = local write "Tab Control"(T1."Hauptansicht" ("Tab Control")) -> ()
          }
          event "Start Button": Value Change {
            n11 = event-data() -> ()  [unwired: 1 in, 1 out]
            n12 = local write "Tab Control"(T1."Hauptansicht" ("Tab Control")) -> ()
          }
          event "Plot_Speichern", "Plot_Speichern 2": Value Change {
            n13 = event-data() -> ()  [unwired: 1 in, 1 out]
            n14 = Select(t=T1."Plotansicht" ("Tab Control"), s="Plot_Speichern 2", f=T1."Hauptansicht" ("Tab Control")) -> (s? t:f=w40:T1)
            n15 = local write "Tab Control"(w40) -> ()
          }
          event "Excel Export": Value Change {
            n16 = event-data() -> ()  [unwired: 1 in, 1 out]
            n17 = local write "Tab Control"(T1."Plotansicht" ("Tab Control")) -> ()
          }
          event "Ansicht_Speichern": Value Change {
            n18 = event-data() -> ()  [unwired: 1 in, 1 out]
            n19 = local write "Tab Control"(T1."Hauptansicht" ("Tab Control")) -> ()
          }
          event "Maximieren": Value Change {
            n20 = event-data() -> ()  [unwired: 1 in, 1 out]
            n21 = local write "Tab Control"(T1."Plotansicht" ("Tab Control")) -> ()
          }
          event "Minimieren": Value Change {
            n22 = event-data() -> ()  [unwired: 1 in, 1 out]
            n23 = local write "Tab Control"(T1."Hauptansicht" ("Tab Control")) -> ()
          }
        }
        n24 = local write "Status"(FALSE ("Status")) -> ()
      }
      frame "Starten der Messung" {
        # "Inidicator für Plotansicht"
        n25 = invoke on="Hystereseschleife und Neukurve" class="XYGraph (strict)" method="Std wiederherstellen"(error in=w95) -> (error out=w94:errorcluster)  [unwired: 2 in, 2 out]
        n26 = Unbundle By Name("GUI Parameter") -> ("Eisenquerschnitt [mm^2]"=w88:dbl, "Wirksame Länge [cm]"=w87:dbl, "Primärwindungszahl"=w86:dbl, "Sekundärwindungszahl"=w85:dbl, "Messwiderstand [Ohm]"=w74:dbl, "Spannungsteilerverhaeltnis (1/x)"=w84:dbl, "Probenbezeichnung"=→"Probenbezeichnung":string, "Dichte des Eisens [g/cm^3]"=→"Dichte des Eisens [g/cm^3]":dbl, "magn. Flussdichte [T]"=→"magn. Flussdichte [T]":dbl, "Frequenz [Hz]"=→"Frequenz [Hz]":dbl, "Namen"=→"Namen":string, "Gruppe"=→"Gruppe":string)
        "Eisenquerschnitt [mm^2]" <- w88
        "Wirksame Länge [cm]" <- w87
        "Primärwindungszahl" <- w86
        "Sekundärwindungszahl" <- w85
        "Messwiderstand [Ohm]" <- w74
        "Spannungsteilerverhältnis (1/x)" <- w84
        n27 = invoke on="Hystereseschleife und Neukurve / Preview" class="XYGraph (strict)" method="Std wiederherstellen"(error in=w94) -> (error out=w77:errorcluster)  [unwired: 2 in, 2 out]
        n28 = Divide(x=w85, y=w84) -> (x/y=w68:dbl)
        "Theo. Primärwindungszahl" <- w68
        n29 = Multiply(x=100.0, y=w86) -> (x*y=w90:dbl)
        n30 = Multiply(x=w87, y=w74) -> (x*y=w89:dbl)
        n31 = Multiply(x=w88, y=w68) -> (x*y=w92:dbl)
        n32 = Divide(x=w90, y=w89) -> (x/y=w66:dbl)
        "Faktor2" <- w66
        n33 = Divide(x=1000000.0, y=w92) -> (x/y=w67:dbl)
        "Faktor1" <- w67
        n34 = Bundle By Name(cluster=w75, "GUI Einstellungen.Minimale Spannung FG"="Minimale Spannung [V]", "Messung Neukurve.Anzahl Messpunkte Neukurve"="Anzahl Messpunkte Neukurve", "Messung Neukurve.Neukurve Messen?"="Neukurve Messen?", "GUI data"="GUI Parameter", "GUI Einstellungen.Anzahl der Messpunkte"="Anzahl der Oszi-Messpunkte", "GUI Einstellungen.VISA Name Oszilloscope"="VISA Name Oszilloscope", "GUI Einstellungen.Maximale Spannung FG"="Maximale Spannung [V]", "GUI Einstellungen.VISA Name Frequenzgenerator"="VISA Name Frequenzgen.", "GUI Einstellungen.Faktor1"=w67, "GUI Einstellungen.Faktor2"=w66, "GUI Einstellungen.Theoretische Primärwindungszahl"=w68) -> (w76:T3)
        n35 = local write "Status"(TRUE ("Status")) -> ()
      }
      frame "Initialisieren Hardware" {
        w99 = FALSE  # Stop Loop?
        n36 = Unbundle By Name(w105) -> ("GUI Einstellungen.VISA Name Oszilloscope"=w101:refnum<visa-resource-name>, "GUI Einstellungen.VISA Name Frequenzgenerator"=w100:refnum<visa-resource-name>)
        n37 = call "Frequenzgenerator_init.vi"("Error_in"=w104, "VISA Name FG in(FG)"=w100) -> ("Error_out"=w103:errorcluster)  [unwired: 8 in, 1 out]
        n38 = call "Oszilloscope_init.vi"("Error_in"=w103, "VISA Name OZ in(OZ)"=w101) -> ("Error_out"=w102:errorcluster)  [unwired: 8 in, 1 out]
        n39 = local write "Status"(TRUE ("Status")) -> ()
      }
      frame "Flussdichte Einstellen" {
        # "#TODO spg & add als output ueberhaupt verwendet?"
        n40 = Unbundle By Name(w114) -> ("GUI Einstellungen"=w107:T5, "GUI data"=w117:T6, "Globale Variablen"=w116:T7)
        n41 = call "Flussdichte_Anpassen.vi"("Error_in"=w115, "Globale Variablen"=w116, "GUI data"=w117, "GUI Einstellungen"=w107) -> ("Error_out"=w109:errorcluster, "Globale Variablen out"=w110:T7, "GUI data out"=w111:T6, "GUI Einstellungen out"=w112:T5)  [unwired: 2 in, 2 out]
        n42 = Bundle By Name(cluster=w114, "GUI Einstellungen"=w112, "GUI data"=w111, "Globale Variablen"=w110) -> (w113:T3)
        n43 = local write "Status"(TRUE ("Status")) -> ()
      }
      frame "Chk Flussdichte Anpassung" {
        n44 = Unbundle By Name(w126) -> ("GUI Einstellungen"=w128:T5, "Globale Variablen"=w127:T7)
        n45 = call "Anpassungspruefung.vi"("Error_in"=w121, "Globale Variablen"=w127, "GUI Einstellungen"=w128) -> ("Error_out"=w122:errorcluster, "Globale Variablen out"=w123:T7, "GUI Einstellungen out"=w124:T5)  [unwired: 6 in]
        n46 = Bundle By Name(cluster=w126, "GUI Einstellungen"=w124, "Globale Variablen"=w123) -> (w125:T3)
        n47 = local write "Status"(TRUE ("Status")) -> ()
      }
      frame "Messung Hystereseschleife" {
        n48 = Unbundle By Name(w133) -> ("Messung Hystereseschleife"=w139:T8, "GUI Einstellungen"=w142:T5, "GUI data"=w141:T6, "Globale Variablen"=w140:T7)
        n49 = call "Messung_Hystereseschleife.vi"("Messung Hystereseschleife"=w139, "Error_in"=w132, "Globale Variablen"=w140, "GUI data"=w141, "GUI Einstellungen"=w142) -> ("Error_out"=w134:errorcluster, "Globale Variablen out"=w135:T7, "GUI data out"=w136:T6, "GUI Einstellungen out"=w137:T5, "Messung Hystereseschleife out"=w138:T8)  [unwired: 2 in]
        n50 = Bundle By Name(cluster=w133, "Messung Hystereseschleife"=w138, "GUI Einstellungen"=w137, "GUI data"=w136, "Globale Variablen"=w135) -> (w144:T3)
        n51 = local write "Status"(TRUE ("Status")) -> ()
      }
      frame "Entmagnetisieren" {
        n52 = Unbundle By Name(w156) -> ("GUI data.Frequenz [Hz]"=w153:dbl, "GUI Einstellungen.VISA Name Frequenzgenerator"=w152:refnum<visa-resource-name>, "Globale Variablen.spg_abw"=w151:dbl)
        n53 = call "Entmagnetisierung.vi"("Frequenz"=w153, "error in (no error)"=w155, "Spannungs Abweichung"=w151, "VISA Name FG in"=w152) -> ("error out"=w154:errorcluster)  [unwired: 6 in, 1 out]
        n54 = local read "Neukurve Messen?"() -> (w149:bool)
        n55 = local write "Status"(TRUE ("Status")) -> ()
        n56 = Select(t=State."Messung Neukurve" ("(Value Not Used)"), s=w149, f=State."Ausgabe Diagramm" ("(Value Not Used)")) -> (s? t:f=w147:T4)
      }
      frame "Messung Neukurve" {
        n57 = Unbundle By Name(w163) -> ("Messung Neukurve.Anzahl Messpunkte Neukurve"=w159:i8, "GUI Einstellungen.Faktor1"=w160:dbl, "GUI Einstellungen.Faktor2"=w161:dbl, "Globale Variablen.spg_abw"=w166:dbl, "GUI Einstellungen.Maximale Spannung FG"=w165:dbl, "GUI data.Frequenz [Hz]"=w168:dbl, "GUI Einstellungen.Anzahl der Messpunkte"=w169:i32, "GUI Einstellungen.VISA Name Oszilloscope"=w170:refnum<visa-resource-name>, "GUI Einstellungen.VISA Name Frequenzgenerator"=w171:refnum<visa-resource-name>)
        n58 = call "MessungNeukurve.vi"("Spannungs Abweichung"=w166, "maximale Spannung"=w165, "Frequency (1000 Hz)"=w168, "Messpunkte Oszi (6000)"=w169, "VISA Name OZ In (OZ)"=w170, "VISA Name FG in"=w171, "error in"=w173, "faktor2"=w161, "Faktor 1"=w160, "Anzahl Messpunkte Neukurve"=w159) -> ("Output B Array"=w162:dbl[], "Output H Array"=w164:dbl[], "error out"=w172:errorcluster)  [unwired: 13 in, 2 out]
        n59 = Bundle By Name(cluster=w163, "B - Neukurve Array"=w162, "H - Neukurve Array"=w164) -> (w167:T3)
        n60 = local write "Status"(TRUE ("Status")) -> ()
      }
      frame "Messung Kommutierungskurve" {
        # "#TODO In Entmagnetisierung2 umbennen funktioniert nicht"
        n61 = Unbundle By Name(w177) -> ("GUI data.Frequenz [Hz]"=w180:dbl, "GUI Einstellungen.VISA Name Frequenzgenerator"=w181:refnum<visa-resource-name>, "GUI Einstellungen.Spannungsabweichung"=w182:dbl)
        n62 = call "Entmagnetisierung.vi"("Frequenz"=w180, "error in (no error)"=w179, "Spannungs Abweichung"=w182, "VISA Name FG in"=w181) -> ("error out"=w178:errorcluster)  [unwired: 6 in, 1 out]
        n63 = local write "Status"(TRUE ("Status")) -> ()
      }
      frame "Ausgabe Diagramm" {
        w196 = State."Ende"  # Nächster Zustand
        n64 = Unbundle By Name(w191) -> ("Messung Hystereseschleife.H - Hysterese Array"=w190:dbl[], "Messung Hystereseschleife.B - Hysterese Array"=w189:dbl[])
        n65 = Unbundle By Name(w191) -> ("H - Neukurve Array"=w194:dbl[], "B - Neukurve Array"=w193:dbl[], "Messung Hystereseschleife.hys_verluste"=→"Hystereseverluste [W]":dbl)
        n66 = Bundle("H - Hysterese Array"=w190, "B - Hysterese Array"=w189) -> (w188:T9)  [unwired: 1 in]
        n67 = Bundle("H - Neukurve Array"=w194, "B - Neukurve Array"=w193) -> (w192:T10)  [unwired: 1 in]
        n68 = Build Array(w188, w192) -> (→"Hystereseschleife und Neukurve" →"Hystereseschleife und Neukurve / Preview":T11)
        n69 = Get Date/Time In Seconds() -> (seconds since 1Jan1904=→"Datum/Uhrzeit":timestamp)
        n70 = local write "Status"(TRUE ("Status")) -> ()
      }
      frame "Ende" {
        w209 = FALSE  # Stop Loop?
        n71 = Unbundle By Name(w207) -> ("GUI Einstellungen.VISA Name Frequenzgenerator"=w200:refnum<visa-resource-name>, "GUI Einstellungen.VISA Name Oszilloscope"=w201:refnum<visa-resource-name>)
        n72 = call "Ansteuerung_Oszilloscope.vi"("Error_in"=w208, "Eingangs-String"=":SYStEM:LOCK OFF;", "VISA Name OZ in(OZ)"=w201) -> ("Error_out"=w203:errorcluster)  [unwired: 6 in, 2 out]
        n73 = call "Ansteuerung_Frequenzgenerator.vi"("Error_in"=w203, "Eingangs-String"=":OUTP OFF;" ("true string"), "VISA Name FZ in(FZ)"=w200) -> ("Error_out"=w202:errorcluster)  [unwired: 5 in, 2 out]
        n74 = local write "Status"(FALSE ("Status")) -> ()
      }
      frame "Plot aufnehmen" {
        n75 = invoke on="Hystereseschleife und Neukurve" class="XYGraph (strict)" method="Bild lesen"(error in=w215) -> (error out=w214:errorcluster, "image data"=w216:T12)  [unwired: 5 in, 4 out]
        n76 = call <vilib>:"Write PNG File.vi"("error in (no error)"=w214, "image data"=w216) -> ("error out"=w213:errorcluster)  [unwired: 8 in, 1 out]
        n77 = call <vilib>:"General Error Handler.vi"("error in (no error)"=w213) -> ()  [unwired: 10 in, 5 out]
        n78 = local write "Status"(FALSE ("Status")) -> ()
      }
      frame "Ansicht speichern" {
        n79 = invoke on="Tab Control" class="TabCtl (strict)" method="Bild lesen"(error in=w221) -> (error out=w224:errorcluster, "image data"=w223:T12)  [unwired: 5 in, 4 out]
        n80 = call <vilib>:"Write PNG File.vi"("error in (no error)"=w224, "image data"=w223) -> ("error out"=w222:errorcluster)  [unwired: 8 in, 1 out]
        n81 = call <vilib>:"General Error Handler.vi"("error in (no error)"=w222) -> ()  [unwired: 10 in, 5 out]
        n82 = local write "Status"(FALSE ("Status")) -> ()
      }
      frame "Excel Export" {
        n83 = invoke on="Hystereseschleife und Neukurve" class="XYGraph (strikt)" method="Plotdaten in Excel exportieren"(error in=w230, "Plot"=1) -> (error out=w229:errorcluster)  [unwired: 2 in, 3 out]
        n84 = local write "Status"(FALSE ("Status")) -> ()
      }
    }
    n85 = Or(x=w5, y=w7) -> (x .or. y?=w6:bool)
  }
  n86 = disable-structure shown="RUN_TIME_ENGINE==True" {
    disable-tunnel: w1 -> [_ _]
    frame condition #0 (active) {
    }
    frame condition #1 {
      # "Call Quit LabVIEW if running as a built application."
      n87 = Quit LabVIEW() -> ()  [unwired: 1 in]
    }
  }
